vi "Write Success_.vi"(8 "error in (no error)":errorcluster, 10 "Success?":bool=TRUE, 11 "ErrorOrSuccess in":refnum<class "ErrorOrSuccess.lvclass">) -> (0 "error out":errorcluster, 3 "ErrorOrSuccess out":refnum<class "ErrorOrSuccess.lvclass">)   [LabVIEW 2020, in "wamplv.lvlib" / "ErrorOrSuccess.lvclass"]
uses:
  ErrorOrSuccess.lvclass
  ErrorOrSuccess.lvclass/ErrorOrSuccess.ctl
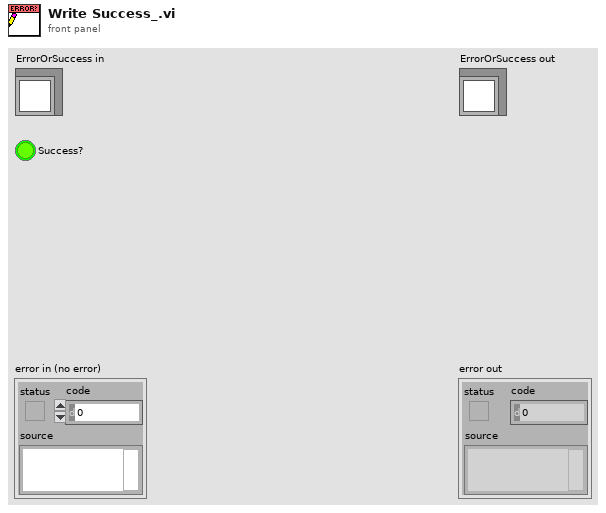
[diagram p1: front panel]
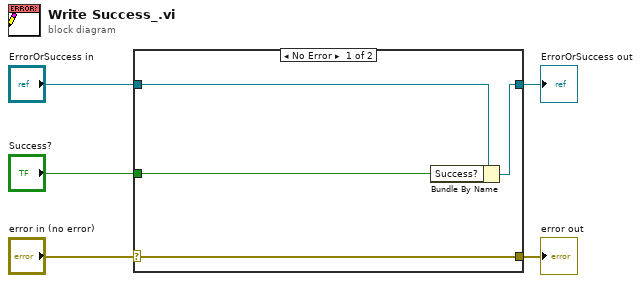
[diagram p0: block diagram]
diagram:
  n1 = case shown="No Error" "error in (no error)" {
    selector: "error in (no error)" -> [w9 w10]
    tunnel: [w9 w10] -> w4
    tunnel: [w7 w11] -> w2
    tunnel: "ErrorOrSuccess in" -> [w8 w11]
    tunnel: "Success?" -> [w6 _]
    frame No Error {
      n2 = Bundle By Name(cluster=w8, "Success?"=w6) -> (w7:refnum<class "ErrorOrSuccess.lvclass">)
    }
    frame Error {
    }
  }
  "error out" <- w4
  "ErrorOrSuccess out" <- w2
